vi "Write Cmd.vi"(8 "error in":errorcluster, 10 "Cmd":string, 11 "SR 3XX HVPS in":refnum<class "SR 3XX HVPS.lvclass">) -> (0 "error out":errorcluster, 3 "SR 3XX HVPS out":refnum<class "SR 3XX HVPS.lvclass">)   [LabVIEW 2014, in "SR 3XX HVPS.lvclass"]
doc: "Basic write on the GPIB port specified by the class. This function simply takes the input string <B>Cmd</B> and appends a new line character and then writes it to the port. If the command is not recognized, an error will be thrown that can be viewed in the Event Status Byte (bit 5 - Command Err)."
uses:
  SR 3XX HVPS.lvclass
  SR 3XX HVPS.lvclass/SR 3XX HVPS.ctl
panel:
  out "appended array":string[](array[string])
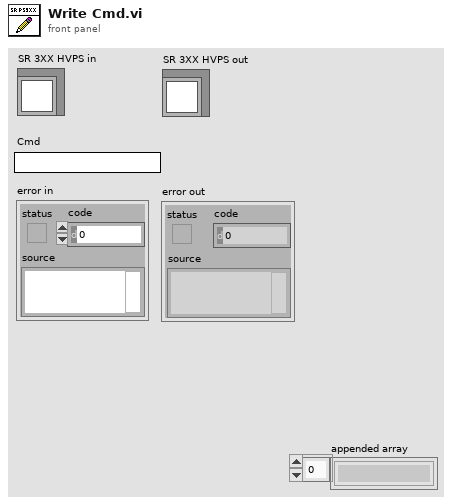
[diagram p1: front panel]
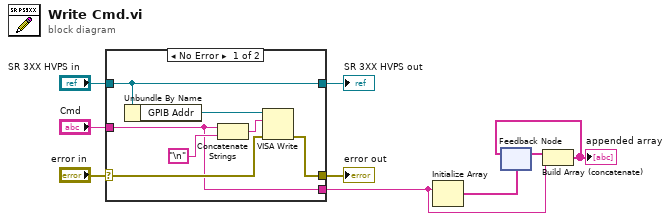
[diagram p0: block diagram]
diagram:
  n1 = case shown="No Error" "error in" {
    selector: "error in" -> [w14 w18]
    tunnel: [w13 w18] -> w8
    tunnel: [w16 w17] -> w6
    tunnel: "SR 3XX HVPS in" -> [w16 w17]
    tunnel: "Cmd" -> [w10 _]
    tunnel: [w10 _] -> w1
    frame No Error {
      n2 = Unbundle By Name(w16) -> ("GPIB Addr"=w15:refnum<visa-resource-name>)
      n3 = Concatenate Strings(w10, "\n") -> (w11:string)
      n4 = VISA Write(VISA resource name=w15, write buffer=w11, error in (no error)=w14) -> (error out=w13:errorcluster)  [unwired: 2 out]
    }
    frame Error {
    }
  }
  "error out" <- w8
  "SR 3XX HVPS out" <- w6
  n5 = Initialize Array(w1) -> (w4:string[])  [unwired: 1 in]
  n6 = feedback #1(w4) -> (w3:string[])
  n7 = Build Array (concatenate)(w3, w1) -> (w2:string[])
  "appended array" <- w2
  n8 = feedback-in #1(w2) -> ()
